vi "oa_Unwrap Wrap Phase in XY Signal (1 Channel).vi"(6 "view":T1={"dB on? (F)"=FALSE, "unwrap phase? (T)"=TRUE, "unit in degree? (T)"=TRUE}, 7 "reset? (F)":bool, 9 "Unwrap?":bool, 11 "XY signal":cluster{"X":dbl[], "Y":dbl[]} {"X" format="%.2f"; "Y" format="%.2f"}) -> (3 "XY signal out":cluster{"X":dbl[], "Y":dbl[]} {"X" format="%.2f"; "Y" format="%.2f"})   [LabVIEW 2017, in "SoundVib_OAUtility.lvlib"]
uses:
  <vilib>/addons/Sound and Vibration/Order Analysis/Utility/SoundVib_OAUtility.lvlib
  <vilib>/addons/Sound and Vibration/Order Analysis/Misc/OAT Convert Phase (1 channel).vi
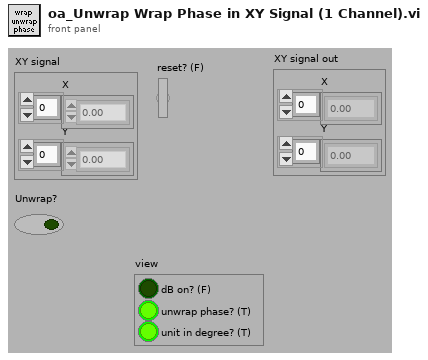
[diagram p1: front panel]
types:
  T1 = cluster{"dB on? (F)":bool, "unwrap phase? (T)":bool, "unit in degree? (T)":bool}
  T2 = cluster{"Unwrap?":bool, "unit in degree? (T)":bool}
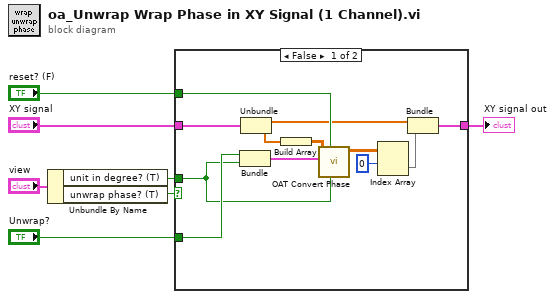
[diagram p0: block diagram]
diagram:
  n1 = Unbundle By Name("view") -> ("unit in degree? (T)"=w3:bool, "unwrap phase? (T)"=w6:bool)
  n2 = case shown="False" w6 {
    tunnel: "XY signal" -> [w19 w20]
    tunnel: [w18 w20] -> w4
    tunnel: w3 -> [w8 _]
    tunnel: "reset? (F)" -> [w17 _]
    tunnel: "Unwrap?" -> [w10 _]
    frame False {
      n3 = Bundle("Unwrap?"=w10, "unit in degree? (T)"=w8) -> (w9:T2)  [unwired: 1 in]
      n4 = Unbundle(w19) -> ("X"=w16:dbl[], "Y"=w15:dbl[])
      n5 = Build Array(w15) -> (w14:dbl[][])
      n6 = call-poly <vilib>:"OAT Convert Phase.vi"("input unit in degree?"=w8, "reset (TRUE)"=w17, "desired phase setting"=w9, "phase in (rad)"=w14) -> ("phase out"=w13:dbl[][])  [unwired: 7 in]
      n7 = Index Array(array=w13, index (row)=0) -> (element=w11:dbl[])  [unwired: 1 in]
      n8 = Bundle("X"=w16, "phase out"=w11) -> (w18:cluster{"X":dbl[], "phase out":dbl[]})  [unwired: 1 in]
    }
    frame True {
    }
  }
  "XY signal out" <- w4
